vi "VI Tree.vi"   [LabVIEW 2011, in "Agilent E5052X.lvlib"]
doc: "This is the instrument driver for the Agilent E5052X. The VI Tree displays all the user-callable VIs of the instrument driver in an organized table."
uses:
  Agilent E5052X.lvlib
  Configure/Configure Measurement Characteristics (Phase Noise).vi
  Configure/Configure Measurement (Phase Noise).vi
  Configure/Configure Sweep (Noise).vi
panel:
  # "(c) 2007-2015 National Instruments.  ALL RIGHTS RESERVED."
  # "SEE DIAGRAM\nFOR VI TREE."
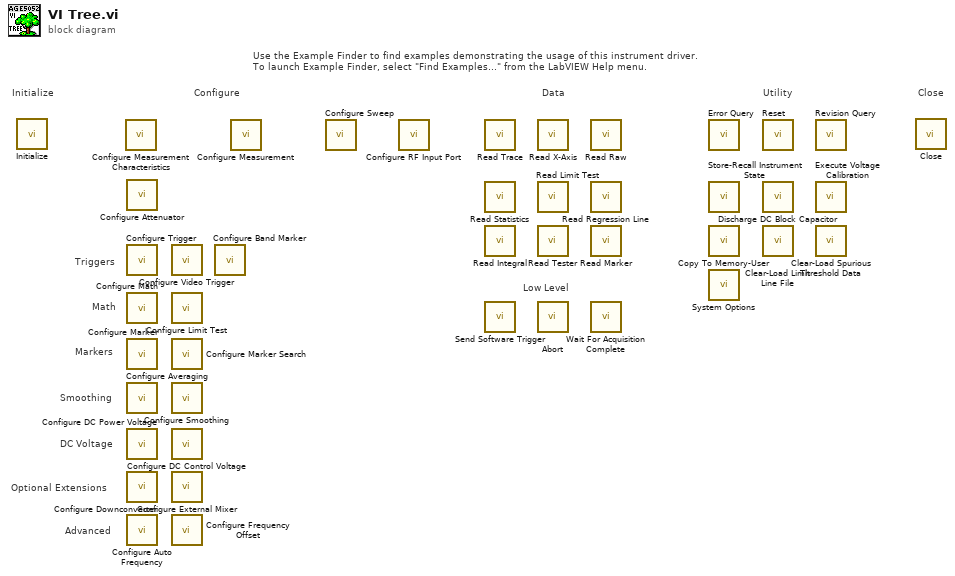
[diagram p0: block diagram]
diagram:
  # "Advanced"
  # "Optional Extensions"
  # "DC Voltage"
  # "Smoothing"
  # "Markers"
  # "Math"
  # "Triggers"
  # "Low Level"
  # "Use the Example Finder to find examples demonstrating the usage of this instrument driver.\nTo launch Example Finder, select \"Find Examples...\" from the LabVIEW Help menu."
  # "Configure"
  # "Utility"
  # "Data"
  # "Close"
  # "Initialize"
  n1 = call "Initialize.vi"() -> ()  [unwired: 10 in, 2 out]
  n2 = call-poly "Configure Measurement Characteristics.vi"() -> ()  [unwired: 14 in, 2 out]
  n3 = call "Configure Attenuator.vi"() -> ()  [unwired: 10 in, 2 out]
  n4 = call "Configure Trigger.vi"() -> ()  [unwired: 14 in, 2 out]
  n5 = call "Configure Math.vi"() -> ()  [unwired: 14 in, 2 out]
  n6 = call "Configure Marker.vi"() -> ()  [unwired: 14 in, 2 out]
  n7 = call "Configure Averaging.vi"() -> ()  [unwired: 10 in, 2 out]
  n8 = call "Configure DC Power Voltage.vi"() -> ()  [unwired: 14 in, 2 out]
  n9 = call "Configure Downconverter.vi"() -> ()  [unwired: 10 in, 2 out]
  n10 = call "Configure Auto Frequency.vi"() -> ()  [unwired: 14 in, 2 out]
  n11 = call "Configure Video Trigger.vi"() -> ()  [unwired: 14 in, 2 out]
  n12 = call "Configure Limit Test.vi"() -> ()  [unwired: 10 in, 2 out]
  n13 = call "Configure Marker Search.vi"() -> ()  [unwired: 14 in, 2 out]
  n14 = call "Configure Smoothing.vi"() -> ()  [unwired: 10 in, 2 out]
  n15 = call "Configure DC Control Voltage.vi"() -> ()  [unwired: 14 in, 2 out]
  n16 = call "Configure External Mixer.vi"() -> ()  [unwired: 10 in, 2 out]
  n17 = call "Configure Frequency Offset.vi"() -> ()  [unwired: 10 in, 2 out]
  n18 = call "Configure Band Marker.vi"() -> ()  [unwired: 14 in, 2 out]
  n19 = call-poly "Configure Measurement.vi"() -> ()  [unwired: 14 in, 2 out]
  n20 = call-poly "Configure Sweep.vi"() -> ()  [unwired: 14 in, 2 out]
  n21 = call "Configure RF Input Port.vi"() -> ()  [unwired: 10 in, 2 out]
  n22 = call "Read Trace.vi"() -> ()  [unwired: 13 in, 3 out]
  n23 = call "Read Statistics.vi"() -> ()  [unwired: 7 in, 5 out]
  n24 = call "Read Integral.vi"() -> ()  [unwired: 8 in, 8 out]
  n25 = call "Send Software Trigger.vi"() -> ()  [unwired: 10 in, 2 out]
  n26 = call "Read X-Axis.vi"() -> ()  [unwired: 9 in, 3 out]
  n27 = call "Read Limit Test.vi"() -> ()  [unwired: 6 in, 10 out]
  n28 = call "Read Tester.vi"() -> ()  [unwired: 7 in, 5 out]
  n29 = call "Abort.vi"() -> ()  [unwired: 10 in, 2 out]
  n30 = call "Read Raw.vi"() -> ()  [unwired: 9 in, 3 out]
  n31 = call "Read Regression Line.vi"() -> ()  [unwired: 8 in, 4 out]
  n32 = call "Read Marker.vi"() -> ()  [unwired: 12 in, 4 out]
  n33 = call "Wait For Acquisition Complete.vi"() -> ()  [unwired: 10 in, 2 out]
  n34 = call "Error Query.vi"() -> ()  [unwired: 8 in, 4 out]
  n35 = call "Store-Recall Instrument State.vi"() -> ()  [unwired: 10 in, 2 out]
  n36 = call "Copy To Memory-User.vi"() -> ()  [unwired: 10 in, 2 out]
  n37 = call "System Options.vi"() -> ()  [unwired: 10 in, 2 out]
  n38 = call "Reset.vi"() -> ()  [unwired: 10 in, 2 out]
  n39 = call "Discharge DC Block Capacitor.vi"() -> ()  [unwired: 10 in, 2 out]
  n40 = call "Clear-Load Limit Line File.vi"() -> ()  [unwired: 14 in, 2 out]
  n41 = call "Revision Query.vi"() -> ()  [unwired: 8 in, 4 out]
  n42 = call "Execute Voltage Calibration.vi"() -> ()  [unwired: 10 in, 2 out]
  n43 = call "Clear-Load Spurious Threshold Data.vi"() -> ()  [unwired: 10 in, 2 out]
  n44 = call "Close.vi"() -> ()  [unwired: 11 in, 1 out]
